vi "magboard_calibrate_nodes.vi"(10 "No. Nodes":i32=64, 11 "Sensor Readings (PACKET)":i16[](array[numeric])) -> (3 "Sensor Output - Position (mm)":dbl[][](array[numeric]))   [LabVIEW 2018]
uses:
  FGVs/FGV States.ctl
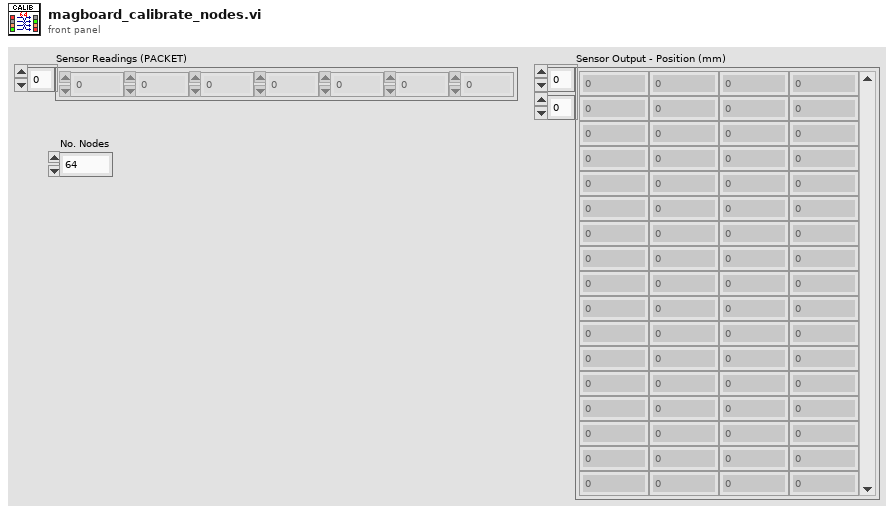
[diagram p1: front panel]
types:
  T1 = typedef "FGV States.ctl" = enum16{"Get", "Set", "Reset"}
  T2 = cluster{cluster{dbl[][], "Array":dbl[][]}, cluster{dbl[][], "Array":dbl[][]}, cluster{dbl[][], "Array":dbl[][]}, cluster{dbl[][], "Array":dbl[][]}}[]
  T3 = cluster{cluster{dbl[][], "Array":dbl[][]}, cluster{dbl[][], "Array":dbl[][]}, cluster{dbl[][], "Array":dbl[][]}, cluster{dbl[][], "Array":dbl[][]}}
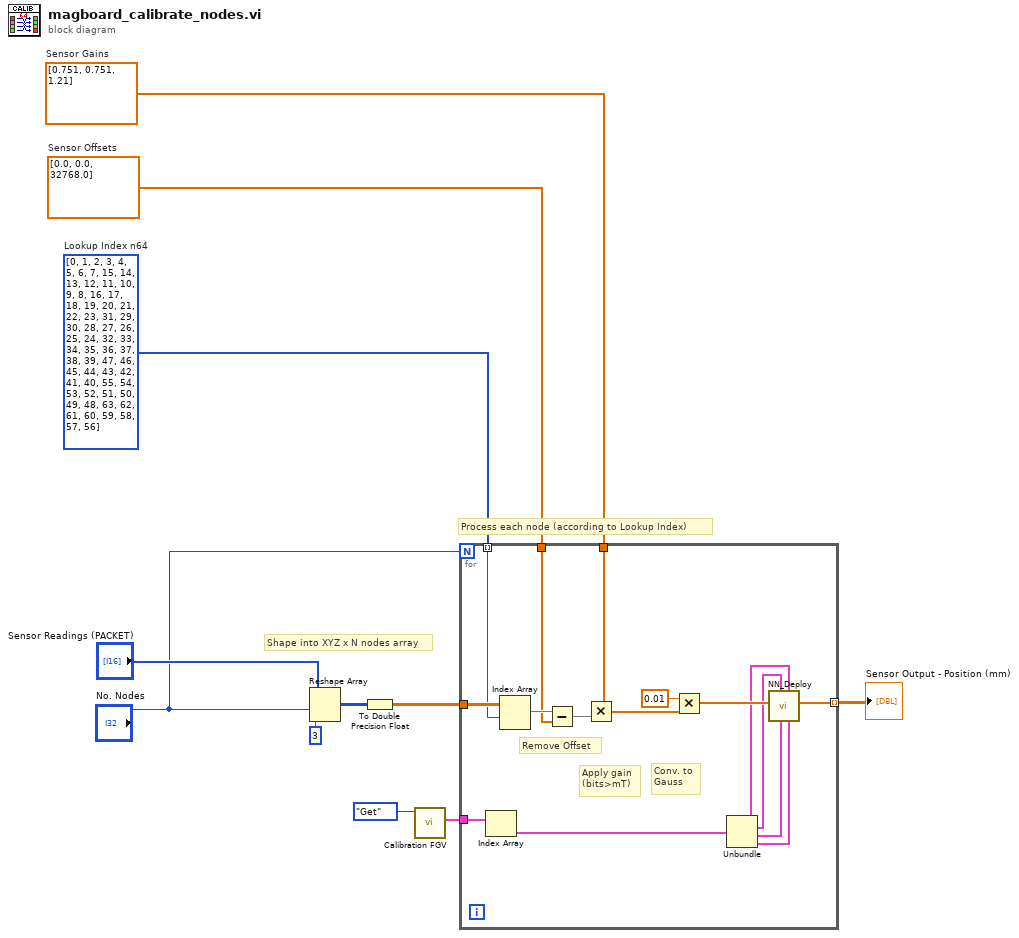
[diagram p0: block diagram]
diagram:
  w5 = dbl[] [0.751, 0.751, 1.21]  # Sensor Gains
  w6 = i32[] [0, 1, 2, 3, 4, 5, 6, 7, 15, 14, 13, 12, 11, 10, 9, 8, 16, 17, 18, 19, 20, 21, 22, 23, 31, 29, 30, 28, 27, 26, 25, 24, 32, 33, 34, 35, 36, 37, 38, 39, 47, 46, 45, 44, 43, 42, 41, 40, 55, 54, 53, 52, 51, 50, 49, 48, 63, 62, 61, 60, 59, 58, 57, 56]  # Lookup Index n64
  w4 = dbl[] [0.0, 0.0, 32768.0]  # Sensor Offsets
  # "Process each node (according to Lookup Index)"
  # "Shape into XYZ x N nodes array"
  n1 = Reshape Array("Sensor Readings (PACKET)", "No. Nodes", 3 ("milliseconds to wait")) -> (w9:i16[][])
  n2 = To Double Precision Float(number=w9) -> (double precision float=w8:dbl[][])
  n3 = call "Calibration FGV.vi"("FGV States"=FGV_States."Get") -> ("Calib in 2"=w2:T2)  [unwired: 10 in]
  n4 = for {
    N: "No. Nodes" -> [_]
    tunnel: w8 -> [w27]
    tunnel: w5 -> [w25]
    tunnel: w6 -> [w24] mode=indexing
    tunnel: w4 -> [w22]
    tunnel: w2 -> [w13]
    tunnel: [w14] -> w1 mode=indexing
    # "Conv. to\nGauss"
    # "Apply gain\n(bits>mT)"
    # "Remove Offset"
    n5 = Index Array(array=w13) -> (element=w12:T3)  [unwired: 1 in]
    n6 = Index Array(array=w27, index (row)=w24) -> (element=w23:dbl[])  [unwired: 1 in]
    n7 = Subtract(x=w23, y=w22) -> (x-y=w26:dbl[])
    n8 = Multiply(x=w25, y=w26) -> (x*y=w20:dbl[])
    n9 = Multiply(x=0.01, y=w20) -> (x*y=w19:dbl[])
    n10 = Unbundle(w12) -> (w18:cluster{dbl[][], "Array":dbl[][]}, w17:cluster{dbl[][], "Array":dbl[][]}, w16:cluster{dbl[][], "Array":dbl[][]}, w15:cluster{dbl[][], "Array":dbl[][]})
    n11 = call "NN_Deploy.vi"("Output Layer"=w15, "Input Layer"=w18, "Layer 2"=w16, "Layer 1"=w17, "Input"=w19) -> ("Output"=w14:dbl[])  [unwired: 6 in]
  }
  "Sensor Output - Position (mm)" <- w1
